vi "Get ID.vi"(11 "Thread in":refnum<class "Thread.lvclass">) -> (2 "ID":i32, 3 "Thread out":refnum<class "Thread.lvclass">)   [LabVIEW 2020, in "DSF Core.lvlib" / "Thread.lvclass"]
uses:
  Thread.lvclass
  Thread.lvclass/Thread.ctl
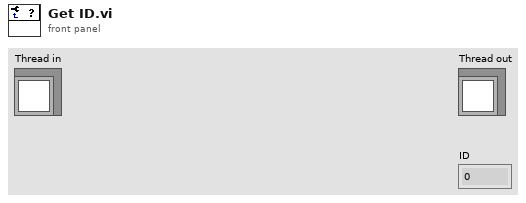
[diagram p1: front panel]
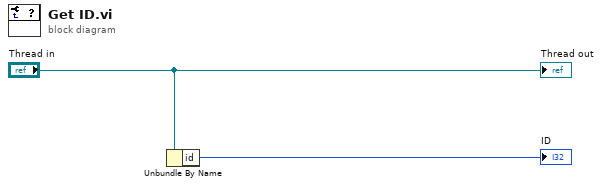
[diagram p0: block diagram]
diagram:
  n1 = Unbundle By Name("Thread in") -> ("id"=→"ID":i32)
  "Thread out" <- "Thread in"
